vi "HelloWorld.vi"() -> ()   [LabVIEW 2015]
panel:
  out "millisecond timer value":u32
  out "Random Number Indicator":dbl
  in  "error in (no error)":cluster{}
  out "Numeric":dbl
  out "number (0 to 1)":dbl
  in  "stop":bool
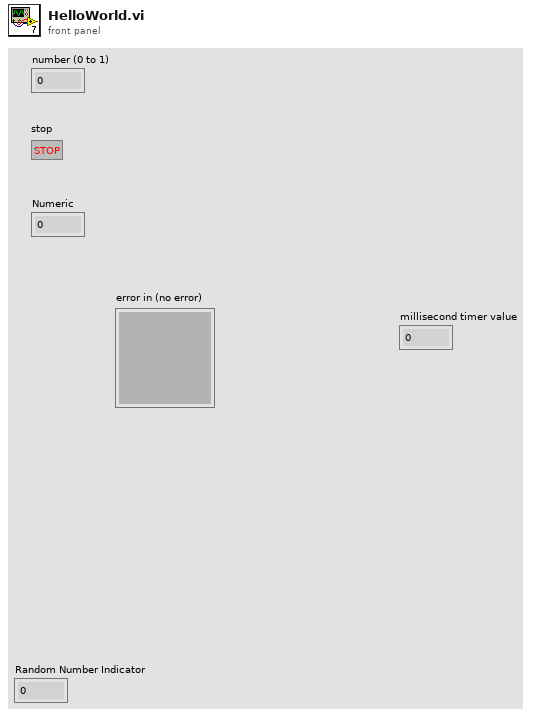
[diagram p1: front panel]
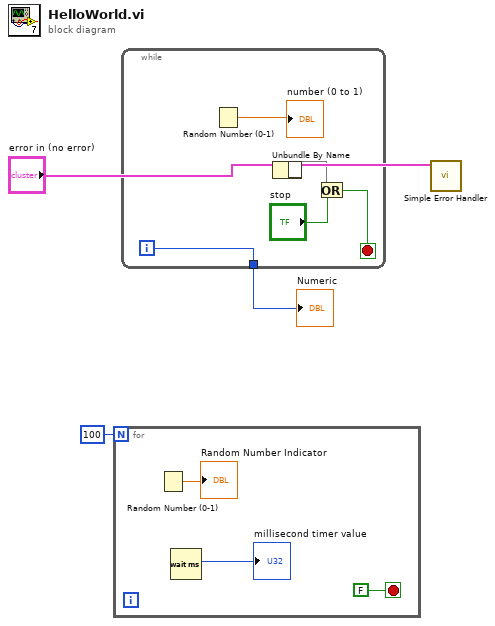
[diagram p0: block diagram]
diagram:
  n1 = for {
    N: 100 -> [_]
    stop <- FALSE stop-if-true
    n2 = Random Number (0-1) ("Random Number")() -> (number: 0 to 1=→"Random Number Indicator":dbl)
    n3 = Wait (ms)() -> (millisecond timer value=→"millisecond timer value":u32)  [unwired: 1 in]
  }
  n4 = while {
    tunnel: [w10] -> w3
    i -> [w10]
    stop <- w9 stop-if-true
    n5 = Random Number (0-1)() -> (number: 0 to 1=→"number (0 to 1)":dbl)
    n6 = Unbundle By Name() -> (w7)  [unwired: 1 in]
    n7 = Or(x=w7, y="stop") -> (x .or. y?=w9:bool)
  }
  "Numeric" <- w3
  n8 = call <vilib>:"Simple Error Handler.vi"("error code (no error:0)"="error in (no error)") -> ()  [unwired: 4 in, 5 out]
